vi "Vicon_Receiver.vi"() -> ()   [LabVIEW 2015]
uses:
  <vilib>/Utility/tcp.llb/UDP Multicast Read-Only Open.vi
panel:
  in  "Tab Control":enum32{"Charts"}(tab)
  out "Translation":dbl[][](graph)
  out "y":dbl
  out "z":dbl
  out "x":dbl
  in  "Stop":bool
  out "roll":dbl
  out "pitch":dbl
  out "yaw":dbl
  out "Rotation":dbl[][](graph)
  out "error out":errorcluster
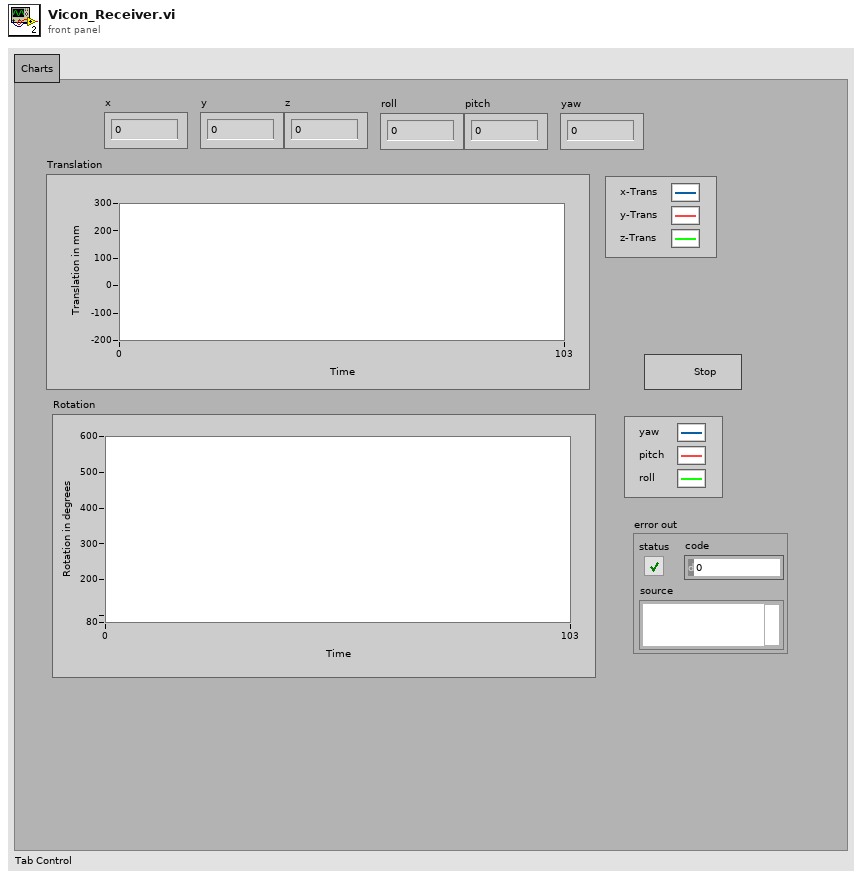
[diagram p1: front panel]
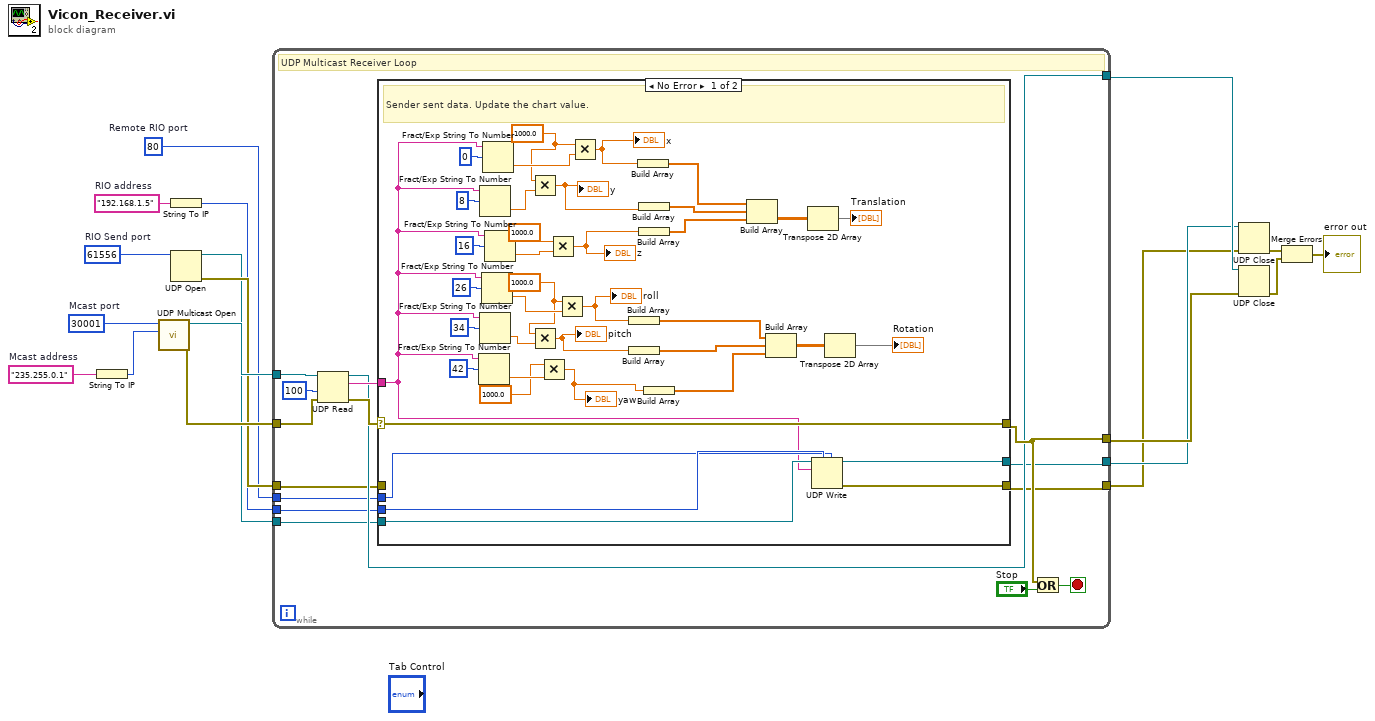
[diagram p0: block diagram]
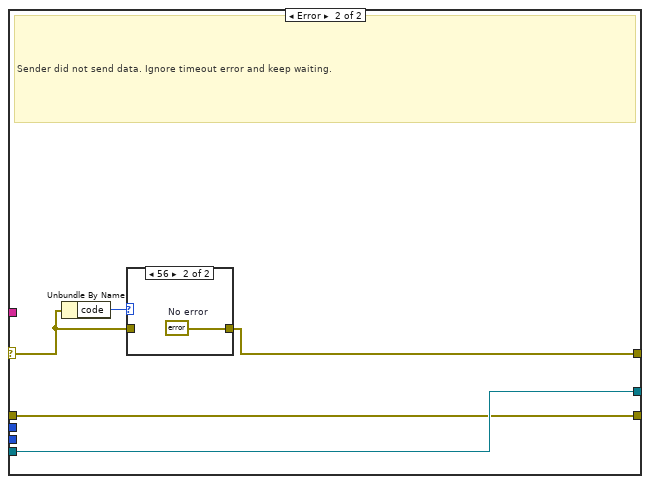
[diagram p2: hidden frame]
diagram:
  w6 = u16 80  # Remote RIO port
  w10 = u16 61556  # RIO Send port
  w11 = "192.168.1.5"  # RIO address
  w13 = u16 30001  # Mcast port
  w17 = "235.255.0.1"  # Mcast address
  n1 = String To IP(1:w17) -> (0:w12:u32)
  n2 = call-poly <vilib>:"UDP Multicast Open.vi"("multicast addr"=w12, "port"=w13) -> ("error out"=w15:errorcluster, "connection ID"=w14:refnum<k16>)  [unwired: 7 in, 1 out]
  n3 = String To IP(1:w11) -> (0:w7:u32)
  n4 = UDP Open(11:w10) -> (port=w8:refnum<k16>, 0:w9:errorcluster)  [unwired: 4 in, 1 out]
  n5 = while {
    tunnel: w14 -> [w33]
    tunnel: [w25] -> w18
    tunnel: w15 -> [w30]
    tunnel: [w26] -> w16
    tunnel: w9 -> [w19]
    tunnel: w8 -> [w24]
    tunnel: w7 -> [w23]
    tunnel: w6 -> [w22]
    tunnel: [w21] -> w5
    tunnel: [w20] -> w4
    stop <- w31 stop-if-true
    # "UDP Multicast Receiver Loop"
    n6 = UDP Read(connection ID=w33, timeout ms (25000)=100, 8:w30) -> (data out=w28:string, error out=w27:errorcluster, 3:w25:refnum<k16>)  [unwired: 3 out]
    n7 = case shown="No Error" w27 {
      selector: w27 -> [w67 w76]
      tunnel: w28 -> [w50 _]
      tunnel: [w67 w75] -> w26
      tunnel: w24 -> [w72 w74]
      tunnel: w23 -> [w71 _]
      tunnel: w22 -> [w70 _]
      tunnel: [w69 w74] -> w21
      tunnel: [w68 w73] -> w20
      tunnel: w19 -> [_ w73]
      frame No Error {
        w39 = 1000.0 ("x")
        w47 = 1000.0 ("y")
        # "Sender sent data. Update the chart value."
        n8 = Fract/Exp String To Number(string=w50, offset=42) -> (number=w36:dbl)  [unwired: 2 in, 1 out]
        n9 = Fract/Exp String To Number(string=w50, offset=8) -> (number=w44:dbl)  [unwired: 2 in, 1 out]
        n10 = Fract/Exp String To Number(string=w50, offset=34) -> (number=w38:dbl)  [unwired: 2 in, 1 out]
        n11 = Fract/Exp String To Number(string=w50, offset=26) -> (number=w41:dbl)  [unwired: 2 in, 1 out]
        n12 = Fract/Exp String To Number(string=w50, offset=0) -> (number=w48:dbl)  [unwired: 2 in, 1 out]
        n13 = Fract/Exp String To Number(string=w50, offset=16) -> (number=w46:dbl)  [unwired: 2 in, 1 out]
        n14 = Multiply(x=w47, y=w44) -> (x*y=w43:dbl)
        "y" <- w43
        n15 = Multiply(x=w39, y=w38) -> (x*y=w37:dbl)
        "pitch" <- w37
        n16 = Multiply(x=1000.0, y=w36) -> (x*y=w34:dbl)
        "yaw" <- w34
        n17 = Multiply(x=1000.0, y=w46) -> (x*y=w42:dbl)
        "z" <- w42
        n18 = Multiply(x=w39, y=w41) -> (x*y=w40:dbl)
        "roll" <- w40
        n19 = Multiply(x=w47, y=w48) -> (x*y=w49:dbl)
        "x" <- w49
        n20 = Build Array(w40) -> (w53:dbl[])
        n21 = Build Array(w37) -> (w54:dbl[])
        n22 = Build Array(w49) -> (w57:dbl[])
        n23 = Build Array(w43) -> (w56:dbl[])
        n24 = Build Array(w42) -> (w61:dbl[])
        n25 = Build Array(w34) -> (w55:dbl[])
        n26 = Build Array(w57, w56, w61) -> (w63:dbl[][])
        n27 = Build Array(w53, w54, w55) -> (w52:dbl[][])
        n28 = Transpose 2D Array(2D array=w63) -> (transposed array=→"Translation":dbl[][])
        n29 = UDP Write(address=w71, port or service name=w70, connection ID=w72, data in=w50) -> (error out=w68:errorcluster, 3:w69:refnum<k16>)  [unwired: 2 in]
        n30 = Transpose 2D Array(2D array=w52) -> (transposed array=→"Rotation":dbl[][])
      }
      frame Error {
        # "Sender did not send data. Ignore timeout error and keep waiting."
        n31 = Unbundle By Name(w76) -> ("code"=w77:i32)
        n32 = case shown="56" w77 {
          tunnel: w76 -> [w78 _]
          tunnel: [w78 w79] -> w75
          frame Default {
          }
          frame 56 {
            w79 = errorcluster {"status"=FALSE, "code"=0, "source"=""}  # No error
          }
        }
      }
    }
    n33 = Or(x=w26, y="Stop") -> (x .or. y?=w31:bool)
  }
  n34 = UDP Close(connection ID=w5, 8:w4) -> (error out=w3:errorcluster)  [unwired: 1 out]
  n35 = UDP Close(connection ID=w18, 8:w16) -> (error out=w2:errorcluster)  [unwired: 1 out]
  n36 = Merge Errors(w3, w2) -> (→"error out":errorcluster)
